vi "GetOccupancyBoard.vi"(8 "error in (no error)":errorcluster, 11 "Board in":refnum<class "Board.lvclass">) -> (0 "error out":errorcluster, 2 "Occupancy":bool[][](array[boolean]), 3 "Board out":refnum<class "Board.lvclass">)   [LabVIEW 2015, in "TronviewGame.lvlib" / "Board.lvclass"]
uses:
  Board.lvclass
  Board.lvclass/Board.ctl
  FieldState.ctl
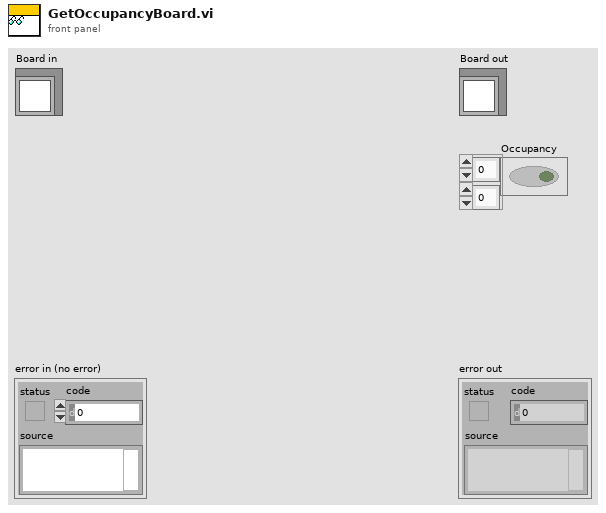
[diagram p1: front panel]
types:
  T1 = typedef "TronviewGame.lvlib/Board.lvclass/FieldState.ctl" = enum16{"Empty", "Blocked", "Player1Position", "Player2Postion", "Player1Marked", "Player2Marked"}
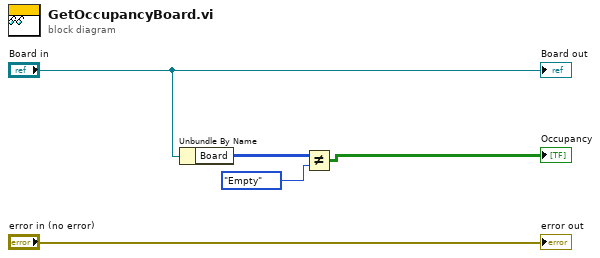
[diagram p0: block diagram]
diagram:
  n1 = Unbundle By Name("Board in") -> ("Board"=w3:T1[][])
  n2 = Not Equal?(x=w3, y=FieldState."Empty" ("FieldState")) -> (x != y?=→"Occupancy":bool[][])
  "error out" <- "error in (no error)"
  "Board out" <- "Board in"
